vi "String Subset.vi"(3 "Offset past End":i32=-1, 4 "Start offset":i32, 5 "JSON":string) -> (1 "substring":string)   [LabVIEW 2020, in "JSONtext.lvlib"]
doc: "String subset between two offsets."
uses:
  <vilib>/JDP Science/JSONtext/JSONtext.lvlib
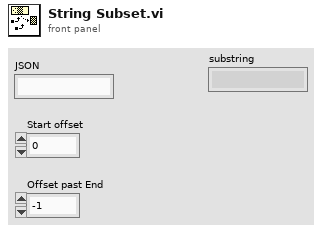
[diagram p1: front panel]
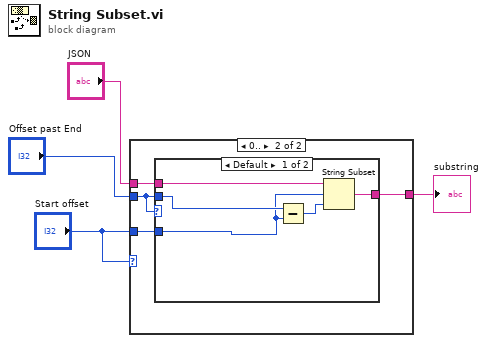
[diagram p0: block diagram]
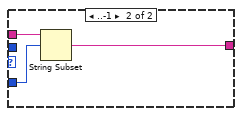
[diagram p3: hidden frame]
diagram:
  n1 = case shown="0.." "Start offset" {
    tunnel: "Offset past End" -> [_ w8]
    tunnel: "JSON" -> [_ w7]
    tunnel: [_ w6] -> w2
    tunnel: "Start offset" -> [_ w5]
    frame ..-1 {
    }
    frame 0.. {
      n2 = case shown="Default" w8 {
        tunnel: w5 -> [w9 w16]
        tunnel: w8 -> [w12 _]
        tunnel: w7 -> [w11 w15]
        tunnel: [w10 w14] -> w6
        frame Default {
          n3 = Subtract(x=w12, y=w9) -> (x-y=w13:i32)
          n4 = String Subset(string=w11, offset (0)=w9, length (rest)=w13) -> (substring=w10:string)
        }
        frame ..-1 {
          n5 = String Subset(string=w15, offset (0)=w16) -> (substring=w14:string)  [unwired: 1 in]
        }
      }
    }
  }
  "substring" <- w2
